vi "sum of n.vi"() -> ()   [LabVIEW 2020]
panel:
  out "Sum":dbl
  in  "Input Number":dbl
  # "Sum of N numbers"
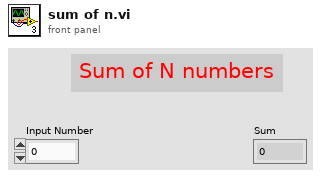
[diagram p1: front panel]
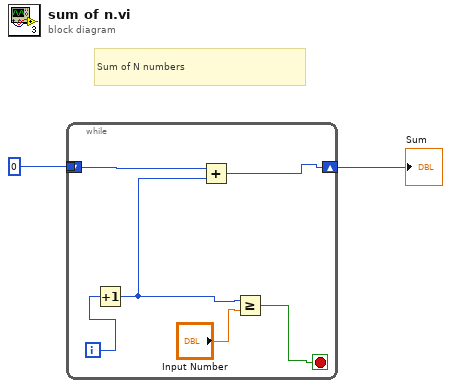
[diagram p0: block diagram]
diagram:
  # "Sum of N numbers"
  n1 = while {
    shift-right: [w7] -> w1
    shift-left: _ -> [w8]
    tunnel: 0 -> [_]
    i -> [w6]
    stop <- w3 stop-if-true
    n2 = Increment(x=w6) -> (x+1=w5:i32)
    n3 = Add(x=w8, y=w5) -> (x+y=w7:i32)
    n4 = Greater Or Equal?(x=w5, y="Input Number") -> (x >= y?=w3:bool)
  }
  "Sum" <- w1
